vi "PrepareHWI.vi"(8 "error in (no error)":errorcluster, 9 "Master Device in":refnum<class "Master Device.lvclass">, 10 "Current Variables":T1[](array[typedef]), 11 "DDS in":refnum<class "DDS.lvclass">) -> (0 "error out":errorcluster, 2 "Master Device out":refnum<class "Master Device.lvclass">, 3 "DDS out":refnum<class "DDS.lvclass">)   [LabVIEW 2013, in "DDS.lvclass"]
uses:
  DDS.lvclass
  Master Device/Master Device.lvclass
  TypeDefs/Active procedure variables.ctl
  DDS.lvclass/DDS.ctl
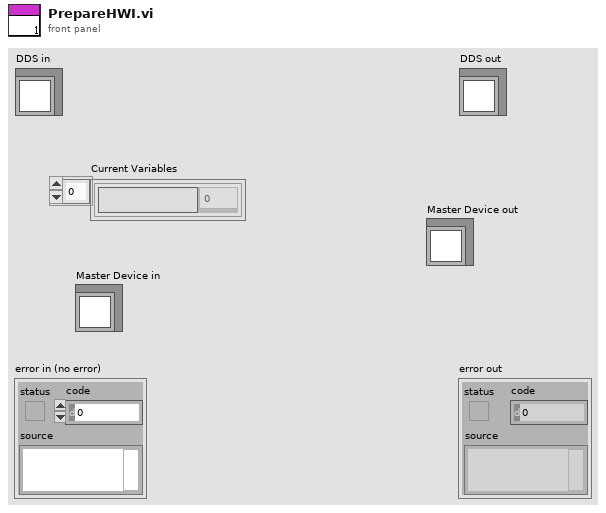
[diagram p1: front panel]
types:
  T1 = typedef "Active procedure variables.ctl" = cluster{"Procedure variable":string, "Value":dbl}
  T2 = cluster{"Triggering":bool[][], "Ramp Info":cluster{"Ramp Index":i32, "Ramp Time":dbl, "Number of Steps":i32}[], "VLIW Array":cluster{"Output Bits":u32, "Data Field":u32, "OP Code":u8, "Delay Count":u64}[]}
  T3 = cluster{"Ramp Index":i32, "Ramp Time":dbl, "Number of Steps":i32}[]
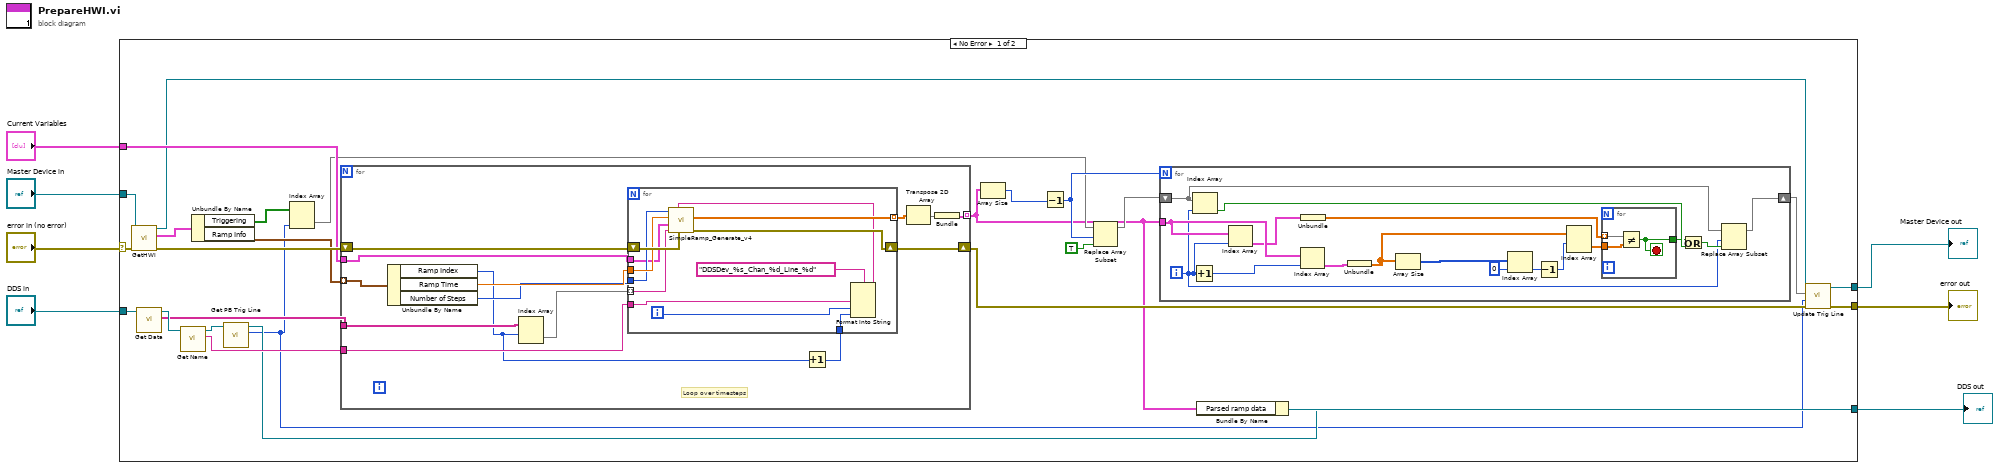
[diagram p0: block diagram]
diagram:
  n1 = case shown="No Error" "error in (no error)" {
    selector: "error in (no error)" -> [w33 w82]
    tunnel: [w23 w81] -> w4
    tunnel: [w22 w82] -> w3
    tunnel: "DDS in" -> [w28 w81]
    tunnel: "Master Device in" -> [w27 w80]
    tunnel: "Current Variables" -> [w26 _]
    tunnel: [w20 w80] -> w1
    frame No Error {
      n2 = call-dynamic "GetHWI.vi"("error in (no error)"=w33, "Master Device in"=w27) -> ("error out"=w32:errorcluster, "Hardware Image"=w31:T2, "Master Device out"=w21:refnum<class "Master Device.lvclass">)  [unwired: 7 in]
      n3 = call-dynamic "Get Data.vi"("Device in"=w28) -> ("Table Indicator"=w24:string[][], "Device out"=w29:refnum<class "DDS.lvclass">)  [unwired: 7 in, 1 out]
      n4 = call-dynamic "Get Name.vi"("Device in"=w29) -> ("Name"=w16:string, "Device out"=w15:refnum<class "DDS.lvclass">)  [unwired: 8 in, 1 out]
      n5 = Unbundle By Name(w31) -> ("Triggering"=w12:bool[][], "Ramp Info"=w30:T3)
      n6 = call-dynamic "Get PB Trig Line.vi"("Device in"=w15) -> ("PB Trigger Line"=w10:u16, "Device out"=w14:refnum<class "DDS.lvclass">)  [unwired: 8 in, 1 out]
      n7 = Index Array(array=w12, index (col)=w10) -> (element=w11:bool[])  [unwired: 1 in]
      n8 = for {
        tunnel: w24 -> [w67]
        shift-right: [w59] -> w13
        shift-left: w32 -> [w66]
        tunnel: w30 -> [w65] mode=indexing
        tunnel: w16 -> [w62]
        tunnel: [w57] -> w8 mode=indexing
        tunnel: w26 -> [w60]
        # "Loop over timesteps"
        n9 = Unbundle By Name(w65) -> ("Ramp Index"=w55:i32, "Ramp Time"=w64:dbl, "Number of Steps"=w63:i32)
        n10 = Index Array(array=w67, index (row)=w55) -> (element=w58:string[])  [unwired: 1 in]
        n11 = Increment(x=w55) -> (x+1=w54:i32)
        n12 = for {
          tunnel: [w79] -> w61 mode=indexing
          tunnel: w58 -> [w71] mode=indexing
          shift-right: [w78] -> w59
          shift-left: w66 -> [w77]
          tunnel: w64 -> [w76]
          tunnel: w63 -> [w75]
          tunnel: w62 -> [w73]
          tunnel: w60 -> [w72]
          tunnel: w54 -> [w69]
          i -> [w68]
          n13 = Format Into String(format string="DDSDev_%s_Chan_%d_Line_%d", w73, w68, w69) -> (resulting string=w70:string)  [unwired: 2 in, 1 out]
          n14 = call "SimpleRamp_Generate_v4.vi"("error in (no error)"=w77, "Error Locator"=w70, "formula"=w71, "Current Variable settings"=w72, "dt"=w76, "Points"=w75) -> ("error out"=w78:errorcluster, "y values"=w79:dbl[])  [unwired: 1 in, 1 out]
        }
        n15 = Transpose 2D Array(2D array=w61) -> (transposed array=w56:dbl[][])
        n16 = Bundle(w56) -> (w57:cluster{dbl[][]})  [unwired: 1 in]
      }
      n17 = Array Size(array=w8) -> (size(s)=w9:i32)
      n18 = Decrement(x=w9) -> (x-1=w17:i32)
      n19 = Replace Array Subset(array=w11, new element=TRUE ("new element/subarray"), index=w17) -> (w18:bool[])
      n20 = for {
        N: w17 -> [_]
        tunnel: w8 -> [w40]
        shift-right: [w41] -> w25
        shift-left: w18 -> [w42]
        i -> [w38]
        n21 = Increment(x=w38) -> (x+1=w39:i32)
        n22 = Index Array(array=w42, index=w38) -> (element=w47:bool)
        n23 = Index Array(array=w40, index=w38) -> (element=w37:cluster{dbl[][]})
        n24 = Index Array(array=w40, index=w39) -> (element=w35:cluster{dbl[][]})
        n25 = Unbundle(w37) -> (w36:dbl[][])
        n26 = Unbundle(w35) -> (w34:dbl[][])
        n27 = Array Size(array=w34) -> (size(s)=w50:i32[])
        n28 = Index Array(array=w50, index=0) -> (element=w45:i32)
        n29 = Decrement(x=w45) -> (x-1=w44:i32)
        n30 = Index Array(array=w34, index (row)=w44) -> (element=w48:dbl[])  [unwired: 1 in]
        n31 = for {
          tunnel: w36 -> [w52] mode=indexing
          tunnel: w48 -> [w53]
          tunnel: [w51] -> w43
          stop <- w51 stop-if-true
          n32 = Not Equal?(x=w52, y=w53) -> (x != y?=w51:bool)
        }
        n33 = Or(x=w43, y=w47) -> (x .or. y?=w46:bool)
        n34 = Replace Array Subset(array=w42, new element=w46, index=w38) -> (w41:bool[])
      }
      n35 = Bundle By Name(cluster=w14, "Parsed ramp data"=w8) -> (w23:refnum<class "DDS.lvclass">)
      n36 = call-dynamic "Update Trig Line.vi"("error in (no error)"=w13, "PB Trigger Line"=w10, "Triggering"=w25, "Master Device in"=w21) -> ("error out"=w22:errorcluster, "Master Device out"=w20:refnum<class "Master Device.lvclass">)  [unwired: 6 in]
    }
    frame Error {
    }
  }
  "error out" <- w3
  "DDS out" <- w4
  "Master Device out" <- w1
